vi "Flush Queue.vi"(8 "error in":errorcluster, 11 "QueueMessageTransport in":refnum<class "QueueMessageTransport.lvclass">) -> (0 "error out":errorcluster, 2 "Remaining Elements":variant[](array[variant]), 3 "QueueMessageTransport out":refnum<class "QueueMessageTransport.lvclass">)   [LabVIEW 2016, in "QueueMessageTransport.lvclass"]
uses:
  QueueMessageTransport.lvclass
  QueueMessageTransport.lvclass/QueueMessageTransport.ctl
panel:
  # "INPUTS"
  # "OUTPUTS"
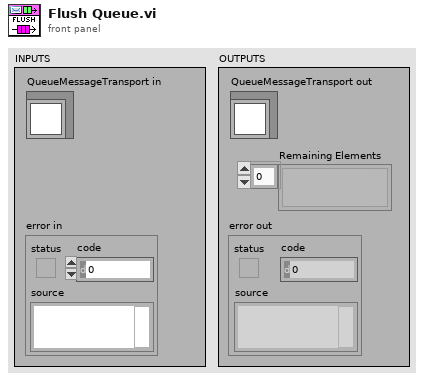
[diagram p1: front panel]
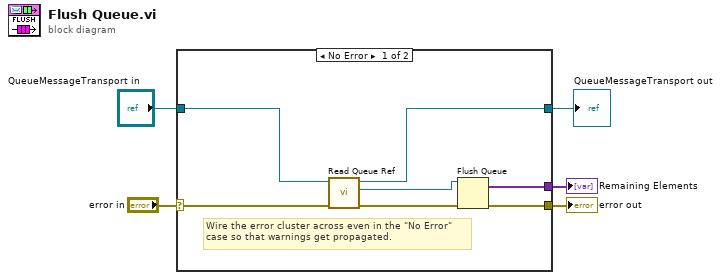
[diagram p0: block diagram]
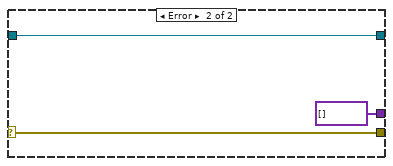
[diagram p2: hidden frame]
diagram:
  n1 = case shown="No Error" "error in" {
    selector: "error in" -> [w12 w15]
    tunnel: [w7 w15] -> w4
    tunnel: [w10 w14] -> w2
    tunnel: "QueueMessageTransport in" -> [w11 w14]
    tunnel: [w6 variant[] [] ("remaining elements")] -> w1
    frame No Error {
      # "Wire the error cluster across even in the \"No Error\"\ncase so that warnings get propagated."
      n2 = call "Read Queue Ref.vi"("error in"=w12, "QueueMessageTransport in"=w11) -> ("error out"=w9:errorcluster, "Queue Ref"=w8:refnum<queue>, "QueueMessageTransport out"=w10:refnum<class "QueueMessageTransport.lvclass">)  [unwired: 7 in]
      n3 = Flush Queue(queue=w8, error in (no error)=w9) -> (remaining elements=w6:variant[], error out=w7:errorcluster)  [unwired: 1 out]
    }
    frame Error {
    }
  }
  "error out" <- w4
  "QueueMessageTransport out" <- w2
  "Remaining Elements" <- w1
